vi "detectPreamble.vi"(1 "data-in":u8[](array[numeric])) -> (0 "detected":bool)   [LabVIEW 2013]
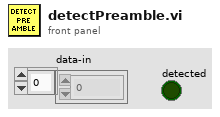
[diagram p1: front panel]
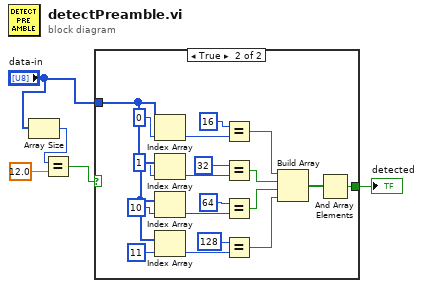
[diagram p0: block diagram]
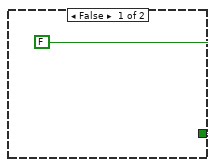
[diagram p2: hidden frame]
diagram:
  n1 = Array Size(array="data-in") -> (size(s)=w3:i32)
  n2 = Equal?(x=w3, y=12.0) -> (x = y?=w2:bool)
  n3 = case shown="True" w2 {
    tunnel: "data-in" -> [_ w25]
    tunnel: [FALSE w7] -> w1
    frame False {
    }
    frame True {
      n4 = Index Array(array=w25, index=0) -> (element=w20:u8)
      n5 = Index Array(array=w25, index=1) -> (element=w18:u8)
      n6 = Index Array(array=w25, index=10) -> (element=w17:u8)
      n7 = Index Array(array=w25, index=11) -> (element=w16:u8)
      n8 = Equal?(x=u8 16, y=w20) -> (x = y?=w9:bool)
      n9 = Equal?(x=u8 32, y=w18) -> (x = y?=w10:bool)
      n10 = Equal?(x=u8 64, y=w17) -> (x = y?=w11:bool)
      n11 = Equal?(x=u8 128, y=w16) -> (x = y?=w12:bool)
      n12 = Build Array(w9, w10, w11, w12) -> (w8:bool[])
      n13 = And Array Elements(Boolean array=w8) -> (logical AND=w7:bool)
    }
  }
  "detected" <- w1
